vi "添加数据.vi"(6 "测试数据":dbl[][](array[numeric]), 8 "错误输入（无错误）":errorcluster, 11 "添加数据":dbl[][](array[numeric])) -> (0 "错误输出":errorcluster, 4 "测试数据输出":dbl[][](array[numeric]))   [LabVIEW 2021]
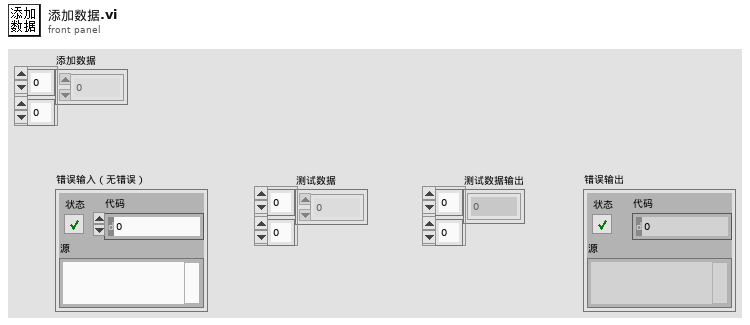
[diagram p1: front panel]
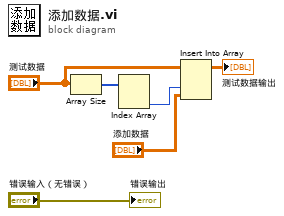
[diagram p0: block diagram]
diagram:
  n1 = Array Size(array="测试数据") -> (size(s)=w6:i32[])
  n2 = Index Array(array=w6) -> (element #2=w5:i32)  [unwired: 2 in, 1 out]
  n3 = Insert Into Array(array="测试数据", index (col)=w5, new element="添加数据") -> (→"测试数据输出":dbl[][])  [unwired: 1 in]
  "错误输出" <- "错误输入（无错误）"
